vi "read_mesureament_more_than_one.vi"(0 "VISA resource name":refnum<visa-resource-name>, 1 "Measurement Function (0: Rise Time)":i32(ring) items=["Rise Time", "Fall Time", "Frequency", "Period", "Voltage RMS(AC)", "Voltage RMS(DC)", "Voltage RMS (AC,cycle)", "Voltage RMS (DC,cycle)", "Voltage Max", "Voltage Min", "Voltage Middle", "Voltage Vpp", "Voltage High", "Voltage Low", "Voltage Average", "Voltage Average (cycle)", "Width Negative", "Width Positive", "Duty Cycle Positive", "Amplitude", "Overshoot", "Preshoot", "Voltage Base", "Voltage Upper", "Time Max", "Time Min", "Color Grade Crossing", "Color Grade Eye Width", "Color Grade Eye Height", "Color Grade Eye Q-Factory", "Color Grade Eye Duty Cycle Distortion(Percent)", "Color Grade Eye Duty Cycle Distortion(Time)", "Color Grade Eye Jitter(PP)", "Color Grade Eye Width(RMS)", "Cycle-cycle Duty Jitter(Rising)", "Cycle-cycle Duty Jitter(Falling)", "Cycle-cycle Jitter(Rising)", "Cycle-cycle Jitter(Falling)", "Cycle-cycle - Width", "Cycle-cycle + Width", "Date Rate", "Unit Interval", "FFT Delta Frequency", "FFT Delta Magnitude", "FFT Frequency", "FFT Magnitude", "Slew Rate", "Area (Entire Display)", "Area(Single Cycle)", "Duty Cycle (Rising)", "Duty Cycle (Falling)"], 5 "Channel (1: Channel 1)":i32(ring)=1 items=["Channel 1"=1, "Channel 2"=2, "Channel 3"=3, "Channel 4"=4, "Function 1"=5, "Function 2"=6, "Function 3"=7, "Function 4"=8, "Memory 1"=9, "Memory 2"=10, "Memory 3"=11, "Memory 4"=12], 7 "Maximum Time (10000ms)":u32=10000, 9 "Channel (1: Channel 1) 2":i32(ring)=5 items=["Channel 1"=1, "Channel 2"=2, "Channel 3"=3, "Channel 4"=4, "Function 1"=5, "Function 2"=6, "Function 3"=7, "Function 4"=8, "Memory 1"=9, "Memory 2"=10, "Memory 3"=11, "Memory 4"=12], 11 "error in (no error)":errorcluster, 12 "Measurement Function (0: Rise Time) 2":i32(ring)=17 items=["Rise Time", "Fall Time", "Frequency", "Period", "Voltage RMS(AC)", "Voltage RMS(DC)", "Voltage RMS (AC,cycle)", "Voltage RMS (DC,cycle)", "Voltage Max", "Voltage Min", "Voltage Middle", "Voltage Vpp", "Voltage High", "Voltage Low", "Voltage Average", "Voltage Average (cycle)", "Width Negative", "Width Positive", "Duty Cycle Positive", "Amplitude", "Overshoot", "Preshoot", "Voltage Base", "Voltage Upper", "Time Max", "Time Min", "Color Grade Crossing", "Color Grade Eye Width", "Color Grade Eye Height", "Color Grade Eye Q-Factory", "Color Grade Eye Duty Cycle Distortion(Percent)", "Color Grade Eye Duty Cycle Distortion(Time)", "Color Grade Eye Jitter(PP)", "Color Grade Eye Width(RMS)", "Cycle-cycle Duty Jitter(Rising)", "Cycle-cycle Duty Jitter(Falling)", "Cycle-cycle Jitter(Rising)", "Cycle-cycle Jitter(Falling)", "Cycle-cycle - Width", "Cycle-cycle + Width", "Date Rate", "Unit Interval", "FFT Delta Frequency", "FFT Delta Magnitude", "FFT Frequency", "FFT Magnitude", "Slew Rate", "Area (Entire Display)", "Area(Single Cycle)", "Duty Cycle (Rising)", "Duty Cycle (Falling)"]) -> (3 "Measurement":dbl, 4 "VISA resource name out":refnum<visa-resource-name>, 6 "Measurement 2":dbl caption="Measurement", 8 "Measurement 3":dbl caption="Measurement", 10 "Measurement 4":dbl caption="Measurement", 14 "Delta Time(s)":dbl, 15 "error out":errorcluster)   [LabVIEW 2009]
uses:
  <instrlib>/Agilent 8000 Series/Public/Data/Low Level/Fetch Measurement (Delta Time).vi
  <instrlib>/Agilent 8000 Series/Public/Data/Low Level/Fetch Measurement (More).vi
  <instrlib>/Agilent 8000 Series/Agilent 8000 Series.lvlib
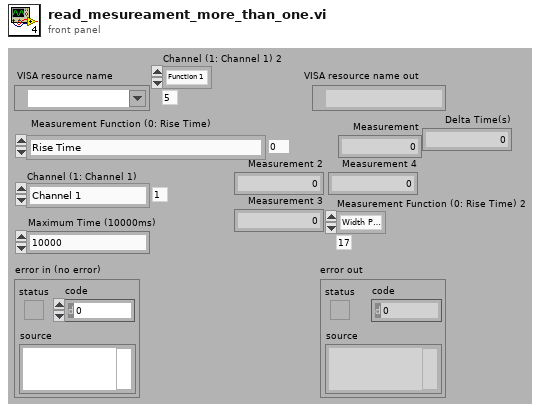
[diagram p1: front panel]
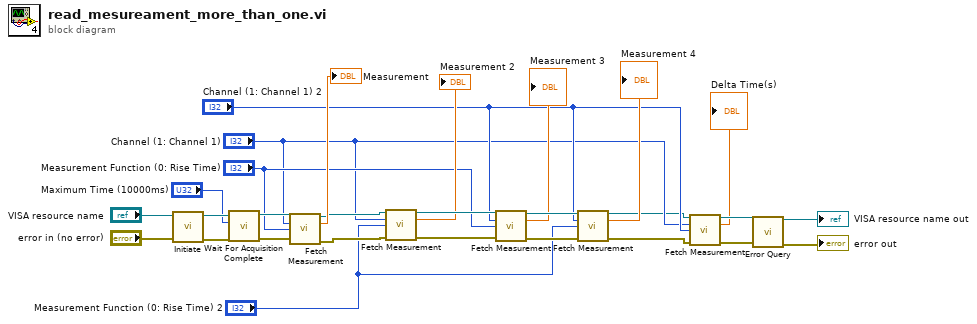
[diagram p0: block diagram]
diagram:
  n1 = call <instrlib>:"Initiate.vi"("error in (no error)"="error in (no error)", "VISA resource name"="VISA resource name") -> ("error out"=w22:errorcluster, "VISA resource name out"=w23:refnum<visa-resource-name>)  [unwired: 8 in]
  n2 = call <instrlib>:"Wait For Acquisition Complete.vi"("error in (no error)"=w22, "Maximum Time (10000ms)"="Maximum Time (10000ms)", "VISA resource name"=w23) -> ("error out"=w21:errorcluster, "VISA resource name out"=w20:refnum<visa-resource-name>)  [unwired: 7 in]
  n3 = call-poly <instrlib>:"Fetch Measurement.vi"("VISA resource name"=w20, "Channel (1: Channel 1)"="Channel (1: Channel 1)", "Measurement Function (0: Rise Time)"="Measurement Function (0: Rise Time)", "error in (no error)"=w21) -> ("VISA resource name out"=w18:refnum<visa-resource-name>, "Measurement"=→"Measurement":dbl, "error out"=w15:errorcluster)  [unwired: 9 in]
  n4 = call-poly <instrlib>:"Fetch Measurement.vi"("VISA resource name"=w18, "Channel (1: Channel 1)"="Channel (1: Channel 1)", "Measurement Function (0: Rise Time)"="Measurement Function (0: Rise Time) 2", "error in (no error)"=w15) -> ("VISA resource name out"=w17:refnum<visa-resource-name>, "Measurement"=→"Measurement 2":dbl, "error out"=w14:errorcluster)  [unwired: 9 in]
  n5 = call-poly <instrlib>:"Fetch Measurement.vi"("VISA resource name"=w17, "Channel (1: Channel 1)"="Channel (1: Channel 1) 2", "Measurement Function (0: Rise Time)"="Measurement Function (0: Rise Time)", "error in (no error)"=w14) -> ("VISA resource name out"=w16:refnum<visa-resource-name>, "Measurement"=→"Measurement 3":dbl, "error out"=w13:errorcluster)  [unwired: 9 in]
  n6 = call-poly <instrlib>:"Fetch Measurement.vi"("VISA resource name"=w16, "Channel (1: Channel 1)"="Channel (1: Channel 1) 2", "Measurement Function (0: Rise Time)"="Measurement Function (0: Rise Time) 2", "error in (no error)"=w13) -> ("VISA resource name out"=w3:refnum<visa-resource-name>, "Measurement"=→"Measurement 4":dbl, "error out"=w4:errorcluster)  [unwired: 9 in]
  n7 = call-poly <instrlib>:"Fetch Measurement.vi"("VISA resource name"=w3, "Channel1 (1: Channel 1)"="Channel (1: Channel 1)", "Channel2 (2: Channel 2)"="Channel (1: Channel 1) 2", "error in (no error)"=w4) -> ("VISA resource name out"=w2:refnum<visa-resource-name>, "Delta Time(s)"=→"Delta Time(s)":dbl, "error out"=w5:errorcluster)  [unwired: 9 in]
  n8 = call <instrlib>:"Error Query.vi"("error in (no error)"=w5, "VISA resource name"=w2) -> ("error out"=→"error out":errorcluster, "VISA resource name out"=→"VISA resource name out":refnum<visa-resource-name>)  [unwired: 6 in, 2 out]
